vi "Init.vi"(8 "error in (no error)":errorcluster, 11 "Simulator in":refnum<class "Simulator.lvclass">) -> (0 "error out":errorcluster, 3 "Simulator out":refnum<class "Simulator.lvclass">)   [LabVIEW 2018, in "Simulator.lvclass"]
uses:
  Simulator.lvclass
  Instrument/Instrument.lvclass
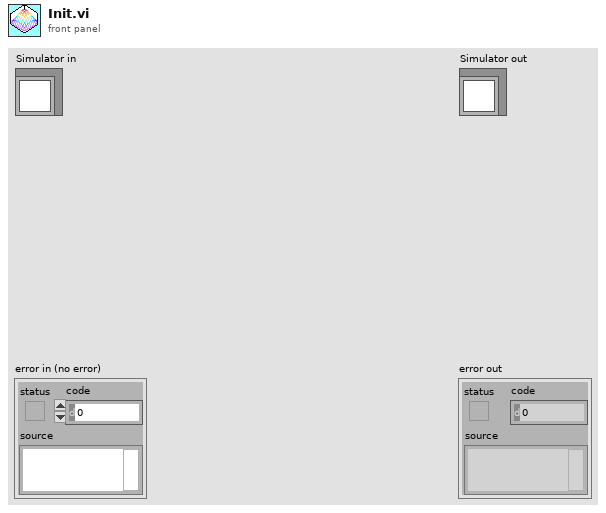
[diagram p1: front panel]
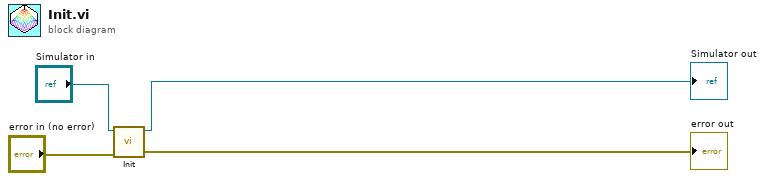
[diagram p0: block diagram]
diagram:
  n1 = call-parent "Init.vi"("error in (no error)"="error in (no error)", "Instrument in"="Simulator in") -> ("error out"=→"error out":errorcluster, "Instrument out"=→"Simulator out":refnum<class "Simulator.lvclass">)  [unwired: 8 in]
